vi "pp2_thread test_subvi.vi"   [LabVIEW 2013]
uses:
  <vilib>/measure/NI_MABase.lvlib
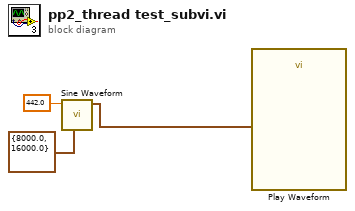
[diagram p0: block diagram]
diagram:
  n1 = call <vilib>:"Sine Waveform.vi"("sampling info"=cluster{"Fs":dbl, "#s":dbl} {"Fs"=8000.0, "#s"=16000.0}, "frequency"=442.0) -> ("signal out"=w1:waveform(dbl))  [unwired: 8 in, 1 out]
  n2 = call "Play Waveform"("Data"=w1) -> ()  [unwired: 18 in, 1 out]
